vi "generate event.vi"(8 "error in":errorcluster, 10 "event":T1, 11 "module in":refnum<class "TBM module execution interface.lvclass">) -> (0 "error out":errorcluster, 2 "failed?":bool, 3 "module out":refnum<class "TBM module execution interface.lvclass">)   [LabVIEW 2013, in "TBM module execution interface.lvclass"]
uses:
  TBM module execution interface.lvclass
  <vilib>/NI/Tag Bus/events/event.ctl
  TBM module execution interface.lvclass/TBM module execution interface.ctl
  <vilib>/NI/Tag Bus/events/data bus events.lvlib
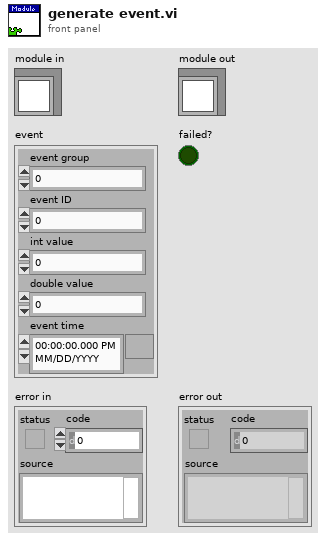
[diagram p1: front panel]
types:
  T1 = typedef "data bus events.lvlib/event.ctl" = cluster{"event group":i64, "event ID":i64, "int value":i64, "double value":dbl, "event time":timestamp}
  T2 = typedef "data bus events.lvlib/event queue.ctl" = cluster{"head":i32, "count":i32, "event array":T1[]}
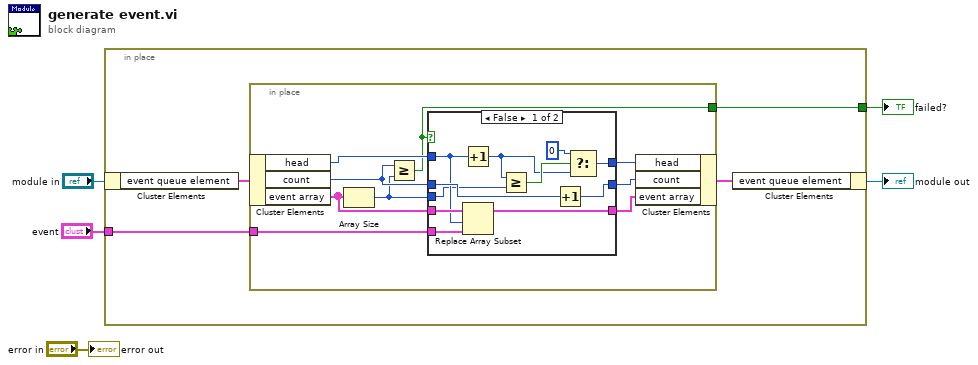
[diagram p0: block diagram]
diagram:
  n1 = in-place {
    in-place-border: "event" -> [w9]
    in-place-border: [w6] -> w1
    n2 = in-place-cluster #1("module in") -> ("event queue element"=w8:T2)
    n3 = in-place {
      in-place-border: w9 -> [w18]
      in-place-border: [w10] -> w6
      n4 = in-place-cluster #2(w8) -> ("head"=w13:i32, "count"=w16:i32, "event array"=w17:T1[])
      n5 = Array Size(array=w17) -> (size(s)=w12:i32)
      n6 = Greater Or Equal?(x=w16, y=w12) -> (x >= y?=w10:bool)
      n7 = case shown="False" w10 {
        tunnel: w18 -> [w27 _]
        tunnel: w17 -> [w29 w31]
        tunnel: w16 -> [w26 w32]
        tunnel: [w25 w32] -> w15
        tunnel: [w28 w31] -> w14
        tunnel: w13 -> [w24 w30]
        tunnel: w12 -> [w22 _]
        tunnel: [w20 w30] -> w11
        frame False {
          n8 = Increment(x=w24) -> (x+1=w21:i32)
          n9 = Replace Array Subset(array=w29, new element=w27, index=w24) -> (w28:T1[])
          n10 = Greater Or Equal?(x=w21, y=w22) -> (x >= y?=w23:bool)
          n11 = Increment(x=w26) -> (x+1=w25:i32)
          n12 = Select(t=0, s=w23, f=w21) -> (s? t:f=w20:i32)
        }
        frame True {
        }
      }
      n13 = in-place-cluster #2("head"=w11, "count"=w15, "event array"=w14) -> (w7:T2)
    }
    n14 = in-place-cluster #1("event queue element"=w7) -> (→"module out":refnum<class "TBM module execution interface.lvclass">)
  }
  "failed?" <- w1
  "error out" <- "error in"
